vi "element_editor_save_as.vi"(10 "Specification Path":refnum<vi>, 11 "Parameters Tree":refnum<vi>) -> ()   [LabVIEW 2019]
uses:
  lib/libSpecValiReader/libSpecValiReader.lvlib
panel:
  # "*******************************************************************\nBiogas Plant Control\n\nAuthor: Paul Zügel\nGCSC-Frankfurt am Main 2020\n\n*******************************************************************"
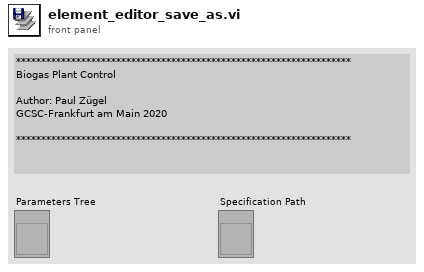
[diagram p1: front panel]
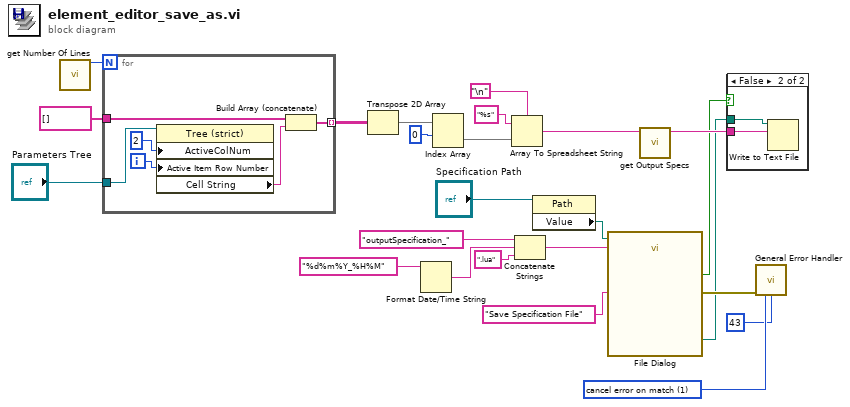
[diagram p0: block diagram]
diagram:
  w10 = 1 items=["no exception", "cancel error on match", "set error on match"] ("[exception action] (none:0)")
  n1 = call "get Number Of Lines.vi"() -> ("function return"=w2:i32)  [unwired: 10 in, 1 out]
  n2 = for {
    N: w2 -> [_]
    tunnel: string[] [] ("Empty Val Arr") -> [w28]
    tunnel: [w27] -> w22 mode=indexing
    tunnel: "Parameters Tree" -> [w25]
    i -> [w30]
    n3 = property on="Property Node" class="Tree (strict)"(reference=w25, "ActiveColNum"=2 ("Active Cell:Active Column Number"), "Active Item Row Number"=w30) -> ("Cell String"=w26:string)  [unwired: 1 in, 2 out]
    n4 = Build Array (concatenate)(w28, w26) -> (w27:string[])
  }
  n5 = Transpose 2D Array(2D array=w22) -> (transposed array=w21:string[][])
  n6 = Format Date/Time String(time format string (%c)="%d%m%Y_%H%M") -> (date/time string=w16:string)  [unwired: 2 in]
  n7 = Index Array(array=w21, index (row)=0) -> (element=w20:string[])  [unwired: 1 in]
  n8 = Array To Spreadsheet String(delimiter (Tab)="\n", array=w20, 3:"%s" ("format string")) -> (spreadsheet string=w4:string)
  n9 = Concatenate Strings("outputSpecification_" ("string"), w16, ".lua" ("string")) -> (w15:string)
  n10 = property class="Path"(reference="Specification Path") -> ("Value"=w5:path)  [unwired: 1 in, 2 out]
  n11 = call "File Dialog"("start path"=w5, "prompt"="Save Specification File", "default name"=w15) -> ("selected path"=w3:path, "cancelled"=w1:bool, "error out"=w14:errorcluster)  [unwired: 9 in, 1 out]
  n12 = call "get Output Specs.vi"("specs"=w4) -> ("output"=w6:string)  [unwired: 9 in, 1 out]
  n13 = case shown="False" w1 {
    tunnel: w6 -> [_ w32]
    tunnel: w3 -> [_ w31]
    frame True {
    }
    frame False {
      n14 = Write to Text File(file (use dialog)=w31, text=w32) -> ()  [unwired: 2 in, 3 out]
    }
  }
  n15 = call <vilib>:"General Error Handler.vi"("error in (no error)"=w14, "[exception action] (none:0)"=w10, "[exception code]"=43) -> ()  [unwired: 8 in, 5 out]
